vi "Association Get All.vi"(8 "error in (no error)":errorcluster, 11 "Connection Refnum":T2) -> (0 "error out":errorcluster, 2 "Associations":T1[](array[typedef]), 3 "Connection Refnum":T2, 4 "Data Present?":bool)   [LabVIEW 2011]
uses:
  Summitek EXT/ODBC/SQL Controls/Connection Refnum.ctl
  Association Record.ctl
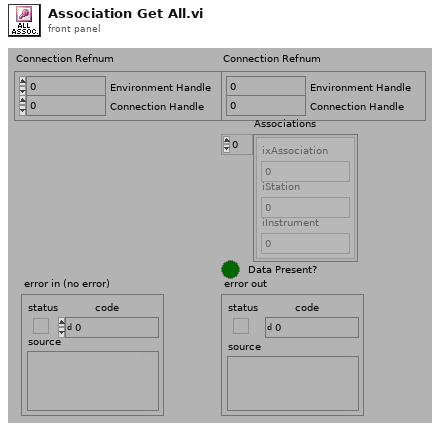
[diagram p1: front panel]
types:
  T1 = typedef "Association Record.ctl" = cluster{"ixAssociation":i32, "iStation":i32, "iInstrument":i32}
  T2 = typedef "Connection Refnum.ctl" = cluster{"Environment Handle":i32, "Connection Handle":i32}
  T3 = typedef "Statement Refnum.ctl" = cluster{"Statement Handle":i32, "Parameter Number":u16}
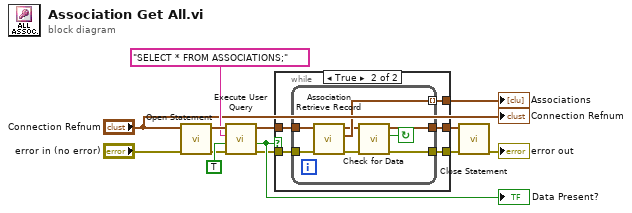
[diagram p0: block diagram]
diagram:
  n1 = call "Open Statement.vi"("error in (no error)"="error in (no error)", "Connection Refnum"="Connection Refnum") -> ("error out"=w6:errorcluster, "Statement Refnum"=w7:T3)  [unwired: 4 out]
  n2 = call "Execute User Query.vi"("error in (no error)"=w6, "Return Data? (f)"=TRUE, "User Query"="SELECT * FROM ASSOCIATIONS;", "Statement Refnum"=w7) -> ("error out"=w12:errorcluster, "Data Present?"=w13:bool, "Statement Refnum"=w11:T3)  [unwired: 1 out]
  "Data Present?" <- w13
  n3 = case shown="True" w13 {
    tunnel: w12 -> [w14 w17]
    tunnel: w11 -> [w15 w16]
    tunnel: [w14 w18] -> w8
    tunnel: [w15 w19] -> w9
    tunnel: [_ w20] -> w3
    frame False {
    }
    frame True {
      n4 = while {
        tunnel: [w28] -> w20 mode=indexing
        tunnel: [w24] -> w19
        tunnel: [w23] -> w18
        tunnel: w17 -> [w22]
        tunnel: w16 -> [w21]
        stop <- w25 continue-if-true
        n5 = call "Association Retrieve Record.vi"("error in (no error)"=w22, "Statement Refnum"=w21) -> ("error out"=w26:errorcluster, "Association"=w28:T1, "Statement Refnum"=w27:T3)  [unwired: 7 out]
        n6 = call "Check for Data.vi"("error in (no error)"=w26, "Statement Refnum"=w27) -> ("error out"=w23:errorcluster, "Data Present?"=w25:bool, "Statement Refnum"=w24:T3)  [unwired: 3 out]
      }
    }
  }
  "Associations" <- w3
  n7 = call "Close Statement.vi"("error in (no error)"=w8, "Statement Refnum"=w9) -> ("error out"=→"error out":errorcluster)  [unwired: 5 out]
  "Connection Refnum" <- "Connection Refnum"
